vi "SwerveJoystickLogic.vi"() -> (2 "Speeds":dbl[](array[numeric]), 3 "Angles":dbl[](array[numeric]))   [LabVIEW 2018]
uses:
  <vilib>/Rock Robotics/Network Tables/NT Read String.vi
  SwerveGlobals.vi
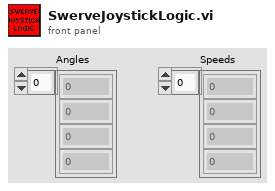
[diagram p1: front panel]
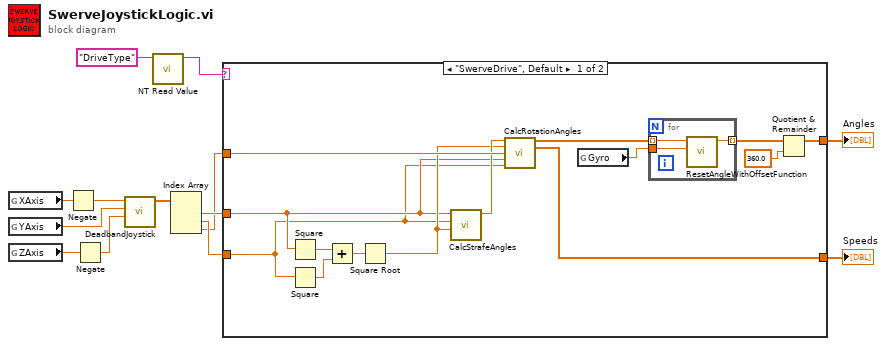
[diagram p0: block diagram]
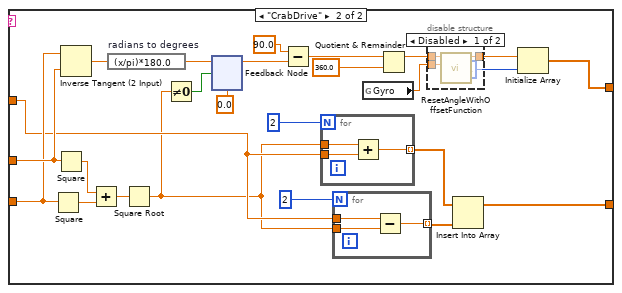
[diagram p2: hidden frame]
diagram:
  n1 = global read "SwerveGlobals.vi" "XAxis"() -> (w9:dbl)
  n2 = global read "SwerveGlobals.vi" "YAxis"() -> (w8:dbl)
  n3 = global read "SwerveGlobals.vi" "ZAxis"() -> (w7:dbl)
  n4 = Negate(x=w9) -> (-x=w2:dbl)
  n5 = Negate(x=w7) -> (-x=w1:dbl)
  n6 = call "DeadbandJoystick.vi"("Z"=w1, "Y"=w8, "X"=w2) -> ("SpeedOutput"=w6:dbl[])  [unwired: 8 in]
  n7 = call-poly <vilib>:"NT Read Value.vi"("Name"="DriveType") -> ("String"=w12:string)  [unwired: 9 in, 1 out]
  n8 = Index Array(array=w6) -> (element #1=w5:dbl, element #2=w4:dbl, element #3=w3:dbl)  [unwired: 3 in]
  n9 = case shown="\"SwerveDrive\", Default" w12 {
    tunnel: w5 -> [w17 w37]
    tunnel: w4 -> [w16 w36]
    tunnel: [w22 w35] -> w11
    tunnel: w3 -> [w23 w34]
    tunnel: [w15 w33] -> w10
    frame "SwerveDrive", Default {
      n10 = Square(x=w17) -> (x^2=w27:dbl)
      n11 = Square(x=w16) -> (x^2=w26:dbl)
      n12 = Add(x=w27, y=w26) -> (x+y=w25:dbl)
      n13 = Square Root(x=w25) -> (sqrt(x)=w18:dbl)
      n14 = call "CalcStrafeAngles.vi"("Speed"=w18, "Y"=w16, "X"=w17) -> ("StrafeAngle"=w19:dbl)  [unwired: 8 in]
      n15 = call "CalcRotationAngles.vi"("StrafeAngle"=w19, "StrafeMagnitude"=w18, "ZAxis"=w23, "XAxis"=w17, "YAxis"=w16) -> ("Angles"=w24:dbl[], "Speeds"=w15:dbl[])  [unwired: 9 in]
      n16 = global read "SwerveGlobals.vi" "Gyro"() -> (w14:dbl)
      n17 = for {
        tunnel: w24 -> [w30] mode=indexing
        tunnel: w14 -> [w29]
        tunnel: [w28] -> w21 mode=indexing
        n18 = call "ResetAngleWithOffsetFunction.vi"("Offset"=w29, "AngleInput"=w30) -> ("AngleOutput"=w28:dbl)  [unwired: 9 in]
      }
      n19 = Quotient & Remainder(x=w21, y=360.0) -> (x-y*floor(x/y)=w22:dbl[])  [unwired: 1 out]
    }
    frame "CrabDrive" {
      n20 = Square(x=w36) -> (x^2=w48:dbl)
      n21 = Square(x=w37) -> (x^2=w49:dbl)
      n22 = Inverse Tangent (2 Input)(1:w37, 2:w36) -> (0:w46:dbl)
      n23 = Add(x=w49, y=w48) -> (x+y=w47:dbl)
      n24 = expression code="(x/pi)*180.0" "radians to degrees"(w46) -> (w43:dbl)
      n25 = Square Root(x=w47) -> (sqrt(x)=w31:dbl)
      n26 = Not Equal To 0?(x=w31) -> (x != 0?=w42:bool)
      n27 = feedback #1(0.0) -> (w32:dbl)
      n28 = feedback-in #1(w43, w42) -> ()
      n29 = Subtract(x=90.0, y=w32) -> (x-y=w45:dbl)
      n30 = for {
        N: 2 -> [_]
        tunnel: w31 -> [w64]
        tunnel: w34 -> [w65]
        tunnel: [w63] -> w52 mode=indexing
        n31 = Add(x=w64, y=w65) -> (x+y=w63:dbl)
      }
      n32 = for {
        N: 2 -> [_]
        tunnel: w31 -> [w60]
        tunnel: w34 -> [w61]
        tunnel: [w62] -> w53 mode=indexing
        n33 = Subtract(x=w61, y=w60) -> (x-y=w62:dbl)
      }
      n34 = global read "SwerveGlobals.vi" "Gyro"() -> (w38:dbl)
      n35 = Quotient & Remainder(x=w45, y=360.0) -> (x-y*floor(x/y)=w39:dbl)  [unwired: 1 out]
      n36 = disable-structure shown="Disabled" {
        disable-tunnel: [w58 w59] -> w40
        disable-tunnel: w39 -> [w57 w59]
        disable-tunnel: w38 -> [w56 _]
        frame Disabled {
          n37 = call "ResetAngleWithOffsetFunction.vi"("Offset"=w56, "AngleInput"=w57) -> ("AngleOutput"=w58:dbl)  [unwired: 9 in]
        }
        frame Enabled {
        }
      }
      n38 = Insert Into Array(array=w52, new element=w53) -> (w33:dbl[])  [unwired: 1 in]
      n39 = Initialize Array(w40, 4 ("dimension size")) -> (w35:dbl[])
    }
  }
  "Angles" <- w11
  "Speeds" <- w10
